vi "Ex2CamNframe.vi"() -> ()   [LabVIEW 2010]
panel:
  in  "Trigger Edge":u32=1 min=1 max=2 step=1
  in  "Trigger Mode":u32=1 min=1 max=6 step=1
  in  "Number of Images":u32=1 min=1 step=1
  in  "ROI":T1={"X start"=1, "X end"=400, "X bin"=1, "Y start"=1, "Y end"=400, "Y bin"=1} {"Y bin" min=1 step=1; "Y end" min=1 step=1; "Y start" min=1 step=1; "X bin" min=1 step=1; "X end" min=1 step=1; "X start" min=1 step=1}
  in  "camera 2 name":string
  in  "camera 1 name":string
  in  "Intensifier Camera 2":bool
  in  "Intensifier Camera 1":bool
  in  "Exposure Camera 2":dbl=0.5 format="%.2f"
  in  "Exposure Camera 1":dbl=0.5 format="%.2f"
  out "error out":errorcluster
  in  "error in (no error)":errorcluster
  # "Ex2CamNframe:\nThis example collects\nfrom two cameras and\nstores in a file. It will\ncollect number of \nimages from each \ncamera"
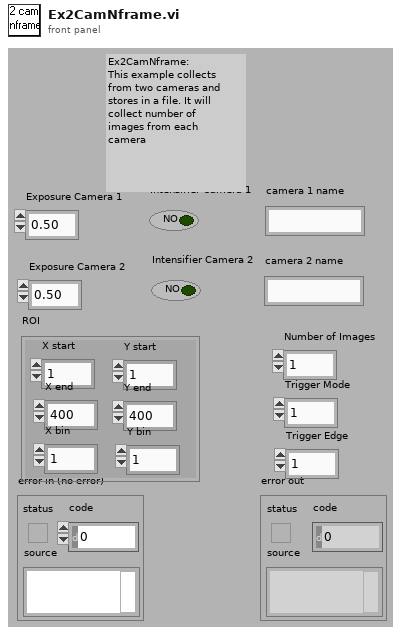
[diagram p1: front panel]
types:
  T1 = cluster{"X start":u32, "X end":u32, "X bin":u32, "Y start":u32, "Y end":u32, "Y bin":u32}
  T2 = cluster{"Camera Handle":u32, "Pulser Handle":u32, "File Handle":u32, "Display Handle":u32, "Image Handle":u32}
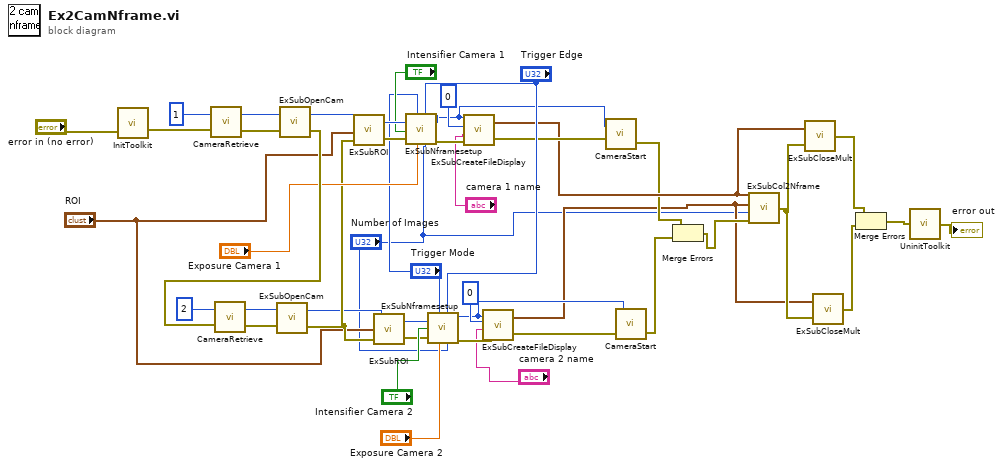
[diagram p0: block diagram]
diagram:
  n1 = call <userlib>:"InitToolkit.vi"("error in"="error in (no error)") -> ("error out"=w37:errorcluster)
  n2 = call <userlib>:"CameraRetrieve.vi"("error in"=w37, "Camera Index"=1) -> ("error out"=w39:errorcluster, "Device ID"=w38:u32)
  n3 = call "ExSubOpenCam.vi"("error in (no error)"=w39, "Camera Device ID"=w38) -> ("error out"=w33:errorcluster, "Camera Handle"=w30:u32)
  n4 = call <userlib>:"CameraRetrieve.vi"("error in"=w33, "Camera Index"=2) -> ("error out"=w34:errorcluster, "Device ID"=w35:u32)
  n5 = call "ExSubOpenCam.vi"("error in (no error)"=w34, "Camera Device ID"=w35) -> ("error out"=w22:errorcluster, "Camera Handle"=w13:u32)
  n6 = call "ExSubROI.vi"("error in (no error)"=w22, "ROI"="ROI", "Camera Handle"=w30) -> ("error out"=w29:errorcluster, "Camera Handle"=w31:u32)
  n7 = call "ExSubROI.vi"("error in (no error)"=w22, "ROI"="ROI", "Camera Handle"=w13) -> ("error out"=w20:errorcluster, "Camera Handle"=w19:u32)
  n8 = call "ExSubNframesetup.vi"("Camera Handle"=w31, "Timing Mode"="Trigger Mode", "Intensifier"="Intensifier Camera 1", "error in (no error)"=w29, "Exposure"="Exposure Camera 1", "Trigger Edge"="Trigger Edge", "Number of Images"="Number of Images") -> ("Camera handle"=w8:u32, "error out"=w26:errorcluster)  [unwired: 2 in]
  n9 = call "ExSubNframesetup.vi"("Camera Handle"=w19, "Timing Mode"="Trigger Mode", "Intensifier"="Intensifier Camera 2", "error in (no error)"=w20, "Exposure"="Exposure Camera 2", "Trigger Edge"="Trigger Edge", "Number of Images"="Number of Images") -> ("Camera handle"=w9:u32, "error out"=w16:errorcluster)  [unwired: 2 in]
  n10 = call "ExSubCreateFileDisplay.vi"("error in (no error)"=w26, "File and Display Name"="camera 1 name", "Pulser Handle"=0, "Camera Handle"=w8) -> ("error out"=w10:errorcluster, "Handles Out"=w7:T2)
  n11 = call "ExSubCreateFileDisplay.vi"("error in (no error)"=w16, "File and Display Name"="camera 2 name", "Pulser Handle"=0, "Camera Handle"=w9) -> ("error out"=w11:errorcluster, "Handles Out"=w2:T2)
  n12 = call <userlib>:"CameraStart.vi"("error in"=w10, "Camera Handle"=w8) -> ("error out"=w4:errorcluster)  [unwired: 1 out]
  n13 = call <userlib>:"CameraStart.vi"("error in"=w11, "Camera Handle"=w9) -> ("error out"=w3:errorcluster)  [unwired: 1 out]
  n14 = Merge Errors(w4, w3) -> (w5:errorcluster)
  n15 = call "ExSubCol2Nframe.vi"("error in (no error)"=w5, "Number of Images"="Number of Images", "Handle Cluster Camera 2"=w2, "Handle Cluster Camera 1"=w7) -> ("error out"=w6:errorcluster)
  n16 = call "ExSubCloseMult.vi"("error in (no error)"=w6, "Handles In"=w7) -> ("error out"=w41:errorcluster)
  n17 = call "ExSubCloseMult.vi"("error in (no error)"=w6, "Handles In"=w2) -> ("error out"=w40:errorcluster)
  n18 = Merge Errors(w41, w40) -> (w43:errorcluster)
  n19 = call <userlib>:"UninitToolkit.vi"("error in"=w43) -> ("error out"=→"error out":errorcluster)
